vi "cmd_set_tip_guard.vi"(8 "error in (no error)":errorcluster, 11 "JSON":string) -> (0 "error out":errorcluster)   [LabVIEW 2021]
doc: "Specifies the tip gurard threshold\n\n :param tg_position: Specifies the z position of the tip when tip guard is triggered\n :param ai_low: Specifies the low threshold for ai (8ch)\n :param fb_low: Specifies the low threshold for feed back (2ch)\n :param ao_low: Specifies the hight threshold for ai (8ch)\n :param fb_high: Specifies the hight threshold for feedback (2ch)"
uses:
  fpga/fpga_dtype_threshold.ctl
  fpga/fpga_dtype_sgl_8ch.ctl
  fpga/fpga_dtype_sgl_fb.ctl
  core/host_global_vars.vi
  <vilib>/Utility/error.llb/Error Cluster From Error Code.vi
  <vilib>/rvi/errors/niLvFpgaAdjustHostInterfaceError.vi
  <vilib>/rvi/interface/nirviReadWriteControl/nirviReadWriteControl.xnode
  FPGA Bitfiles/openlabspm_FPGATarget_fpgamain_eo-gUZR5D1g.lvbitx
  fpga/fpga_main.vi
  NiFpgaLv.dll
panel:
  in  "args":T1
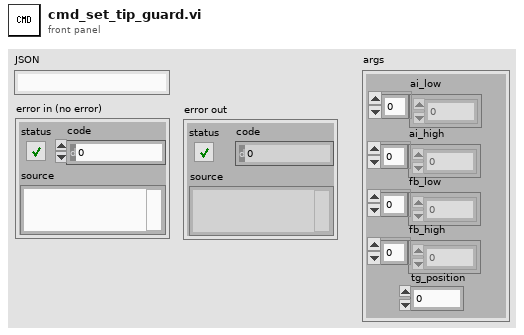
[diagram p1: front panel]
types:
  T1 = cluster{"ai_low":sgl[], "ai_high":sgl[], "fb_low":sgl[], "fb_high":sgl[], "tg_position":dbl}
  T2 = typedef "fpga_dtype_threshold.ctl" = cluster{"ai limit (high)":T3, "fb limit (hight)":T4, "ai limit (low)":T3, "fb limit (low)":T4}
  T3 = typedef "fpga_dtype_sgl_8ch.ctl" = cluster{"ch 0":sgl, "ch 1":sgl, "ch 2":sgl, "ch 3":sgl, "ch 4":sgl, "ch 5":sgl, "ch 6":sgl, "ch 7":sgl}
  T4 = typedef "fpga_dtype_sgl_fb.ctl" = cluster{"fb 0":sgl, "fb 1":sgl}
  T5 = cluster{"ai_low[0]":sgl, "ai_low[1]":sgl, "ai_low[2]":sgl, "ai_low[3]":sgl, "ai_low[4]":sgl, "ai_low[5]":sgl, "ai_low[6]":sgl, "ai_low[7]":sgl}
  T6 = cluster{"ai_high[0]":sgl, "ai_high[1]":sgl, "ai_high[2]":sgl, "ai_high[3]":sgl, "ai_high[4]":sgl, "ai_high[5]":sgl, "ai_high[6]":sgl, "ai_high[7]":sgl}
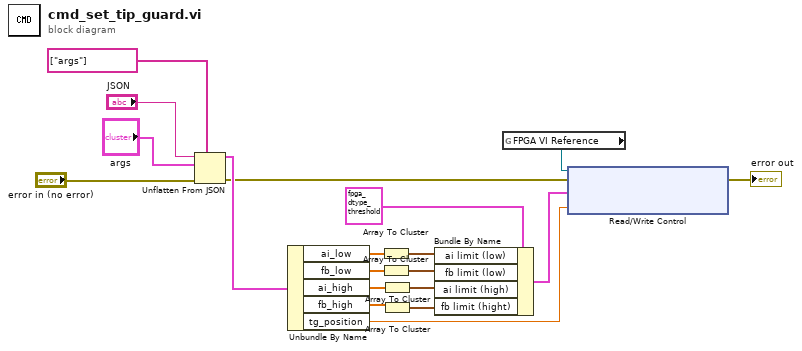
[diagram p0: block diagram]
diagram:
  n1 = Unflatten From JSON(path=string[] ["args"], JSON string="JSON", type and defaults="args", error in (no error)="error in (no error)") -> (value=w13:T1, error out=w2:errorcluster)  [unwired: 3 in]
  n2 = Unbundle By Name(w13) -> ("ai_low"=w11:sgl[], "fb_low"=w5:sgl[], "ai_high"=w7:sgl[], "fb_high"=w9:sgl[], "tg_position"=w1:dbl)
  n3 = Array To Cluster(array=w11) -> (cluster=w10:T5)
  n4 = Array To Cluster(array=w5) -> (cluster=w4:cluster{"fb_low[0]":sgl, "fb_low[1]":sgl})
  n5 = Array To Cluster(array=w7) -> (cluster=w6:T6)
  n6 = Array To Cluster(array=w9) -> (cluster=w8:cluster{"fb_high[0]":sgl, "fb_high[1]":sgl})
  n7 = Bundle By Name(cluster=T2 {"ai limit (high)"={"ch 0"=0.0, "ch 1"=0.0, "ch 2"=0.0, "ch 3"=0.0, "ch 4"=0.0, "ch 5"=0.0, "ch 6"=0.0, "ch 7"=0.0}, "fb limit (hight)"={"fb 0"=0.0, "fb 1"=0.0}, "ai limit (low)"={"ch 0"=0.0, "ch 1"=0.0, "ch 2"=0.0, "ch 3"=0.0, "ch 4"=0.0, "ch 5"=0.0, "ch 6"=0.0, "ch 7"=0.0}, "fb limit (low)"={"fb 0"=0.0, "fb 1"=0.0}} ("threshold"), "ai limit (low)"=w10, "fb limit (low)"=w4, "ai limit (high)"=w6, "fb limit (hight)"=w8) -> (w3:T2)
  n8 = global read "host_global_vars.vi" "FPGA VI Reference"() -> (w14:refnum<k20>)
  n9 = xnode "Read/Write Control"("FPGA VI Reference In"=w14, "error in"=w2, "tip guard"=w3, "tip guard position"=w1) -> ("error out"=→"error out":errorcluster)  [unwired: 1 out]
